vi "9221 4Ch Analog Input.vi"(1 "9221 I/O":T1={"9221 AI0"="NI 9221/AI0", "9221 AI1"="NI 9221/AI1", "9221 AI2"="NI 9221/AI2", "9221 AI3"="NI 9221/AI3"}) -> (0 "Packets":u64[](array[numeric]))   [LabVIEW 2010]
uses:
  <vilib>/eio/EIONode/EIONode.xnode
  <vilib>/rvi/eio/nirviEIOImplementation/nirviEIOImplementation.xnode
  <vilib>/rvi/eio/common/nirviEmuClasses.ctl
  <vilib>/rvi/eio/common/nirviEmuTemplateMethod_noerrors.vi
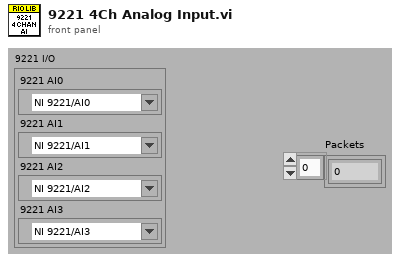
[diagram p1: front panel]
types:
  T1 = cluster{"9221 AI0":refnum<k21>, "9221 AI1":refnum<k21>, "9221 AI2":refnum<k21>, "9221 AI3":refnum<k21>}
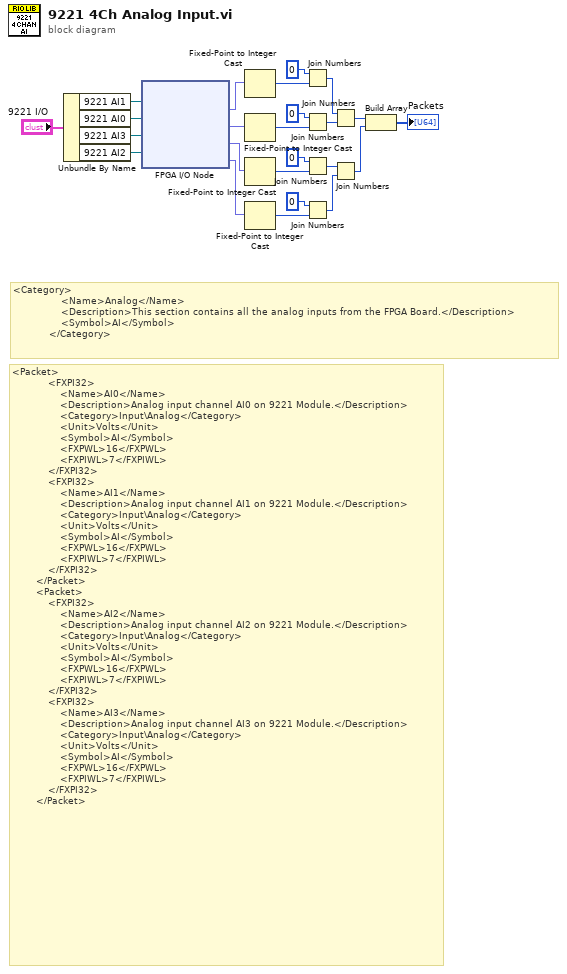
[diagram p0: block diagram]
diagram:
  # "<Category>\n                <Name>Analog</Name>\n                <Description>This section contains all the analog inputs from the FPGA Board.</Description>\n                <Symbol>AI</Symbol>\n            </Category>"
  # "<Packet>\n            <FXPI32>\n                <Name>AI0</Name>\n                <Description>Analog input channel AI0 on 9221 Module.</Description>\n                <Category>Input\\Analog</Category>\n                <Unit>Volts</Unit>\n                <Symbol>AI</Symbol>\n                <FXPWL>16</FXPWL>\n                <FXPIWL>7</FXPIWL>\n            </FXPI32>\n            <FXPI32>\n                <Name>AI1</Name>\n                <Description>Analog input channel AI1 on 9221 Module.</Description>\n                <Category>Input\\Analog</Category>\n                <Unit>Volts</Unit>\n                <Symbol>AI</Symbol>\n                <FXPWL>16</FXPWL>\n                <FXPIWL>7</FXPIWL>\n            </FXPI32>\n        </Packet>\n        <Packet>\n            <FXPI32>\n                <Name>AI2</Name>\n                <Description>Analog input channel AI2 on 9221 Module.</Description>\n                <Category>Input\\Analog</Category>\n                <Unit>Volts</Unit>\n                <Symbol>AI</Symbol>\n                <FXPWL>16</FXPWL>\n                <FXPIWL>7</FXPIWL>\n            </FXPI32>\n            <FXPI32>\n                <Name>AI3</Name>\n                <Description>Analog input channel AI3 on 9221 Module.</Description>\n                <Category>Input\\Analog</Category>\n                <Unit>Volts</Unit>\n                <Symbol>AI</Symbol>\n                <FXPWL>16</FXPWL>\n                <FXPIWL>7</FXPIWL>\n            </FXPI32>\n        </Packet>"
  n1 = Unbundle By Name("9221 I/O") -> ("9221 AI1"=w20:refnum<k21>, "9221 AI0"=w22:refnum<k21>, "9221 AI3"=w21:refnum<k21>, "9221 AI2"=w23:refnum<k21>)
  n2 = xnode "FPGA I/O Node"("FPGA I/O In"=w20, "FPGA I/O In"=w22, "FPGA I/O In"=w21, "FPGA I/O In"=w23) -> ("I/O Item"=w4:fxp<+/-,16,7>, "I/O Item"=w3:fxp<+/-,16,7>, "I/O Item"=w2:fxp<+/-,16,7>, "I/O Item"=w1:fxp<+/-,16,7>)  [unwired: 4 out]
  n3 = Fixed-Point to Integer Cast(1:w4) -> (0:w19:i16)
  n4 = Fixed-Point to Integer Cast(1:w3) -> (0:w16:i16)
  n5 = Fixed-Point to Integer Cast(1:w2) -> (0:w13:i16)
  n6 = Fixed-Point to Integer Cast(1:w1) -> (0:w10:i16)
  n7 = Join Numbers(hi=i16 0, lo=w19) -> ((hi.lo)=w15:u32)
  n8 = Join Numbers(hi=i16 0, lo=w16) -> ((hi.lo)=w14:u32)
  n9 = Join Numbers(hi=i16 0, lo=w13) -> ((hi.lo)=w9:u32)
  n10 = Join Numbers(hi=i16 0, lo=w10) -> ((hi.lo)=w8:u32)
  n11 = Join Numbers(hi=w15, lo=w14) -> ((hi.lo)=w7:u64)
  n12 = Join Numbers(hi=w9, lo=w8) -> ((hi.lo)=w6:u64)
  n13 = Build Array(w7, w6) -> (→"Packets":u64[])
